vi "ExTestMoveSpectroGlbMult.vi"() -> ()   [LabVIEW 2010]
uses:
  GlbCamHndls.vi
panel:
  in  "Spectrometer number":u32=1 min=1 step=1
  in  "Wavelength":dbl format="%.2f"
  in  "Grating Speed":dbl=2000.0 min=1.0 step=1.0 format="%.2f"
  in  "Grating number":i16=1 min=1 max=100 step=1
  out "error out":errorcluster
  in  "error in (no error)":errorcluster
  # "ExTestMoveSpectroGlbMult.vi : this\nsub vi takes the gloabl handles  for\nthe spectrometer and moves the \nspectrometer (grating, speed, \nand wavelength)."
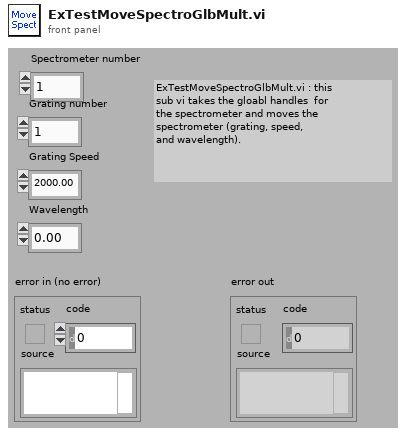
[diagram p1: front panel]
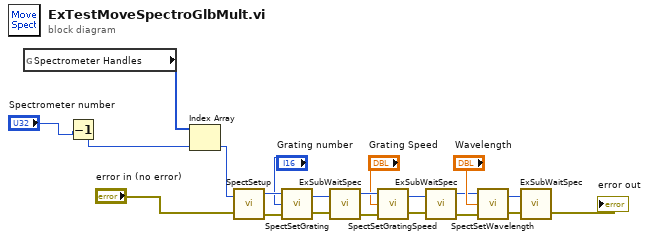
[diagram p0: block diagram]
diagram:
  n1 = global read "GlbCamHndls.vi" "Spectrometer Handles"() -> (w4:u32[])
  n2 = Decrement(x="Spectrometer number") -> (x-1=w5:u32)
  n3 = Index Array(array=w4, index=w5) -> (element=w3:u32)
  n4 = call <userlib>:"SpectSetup.vi"("error in"="error in (no error)", "Spectrometer Handle"=w3) -> ("error out"=w11:errorcluster, "Spectrometer Handle"=w12:u32)
  n5 = call <userlib>:"SpectSetGrating.vi"("error in"=w11, "Grating Number"="Grating number", "Sepctrometer Handle"=w12) -> ("error out"=w18:errorcluster, "Spectrometer Handle"=w17:u32)
  n6 = call "ExSubWaitSpec.vi"("error in (no error)"=w18, "Spectrometer Handle"=w17) -> ("error out"=w16:errorcluster, "Spectrometer handle"=w15:u32)
  n7 = call <userlib>:"SpectSetGratingSpeed.vi"("error in"=w16, "Grating Speed"="Grating Speed", "Spectrometer Handle"=w15) -> ("error out"=w13:errorcluster, "Spectrometer Handle"=w14:u32)
  n8 = call "ExSubWaitSpec.vi"("error in (no error)"=w13, "Spectrometer Handle"=w14) -> ("error out"=w9:errorcluster, "Spectrometer handle"=w10:u32)
  n9 = call <userlib>:"SpectSetWavelength.vi"("error in"=w9, "Wavelength"="Wavelength", "Spectrometer Handle"=w10) -> ("error out"=w21:errorcluster, "Spectrumeter Handle"=w20:u32)
  n10 = call "ExSubWaitSpec.vi"("error in (no error)"=w21, "Spectrometer Handle"=w20) -> ("error out"=→"error out":errorcluster)  [unwired: 1 out]
